vi "Create Channel Name Array.vi"(8 "error in":errorcluster, 9 "Number of Channels":u32=1, 10 "Channel Format String":string, 11 "Plugin Name":string) -> (0 "error out":errorcluster, 2 "Channel Names":string[](array[string]))   [LabVIEW 2023, in "Utilities.lvlib"]
uses:
  Utilities.lvlib
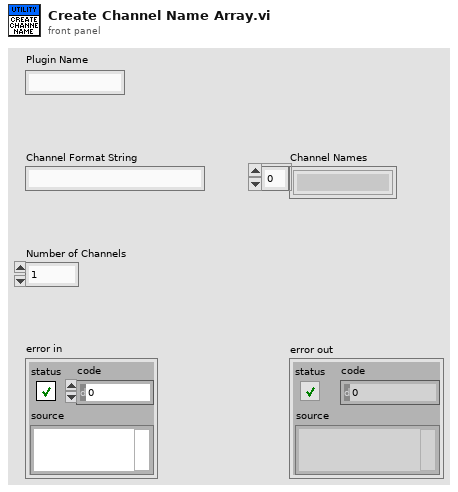
[diagram p1: front panel]
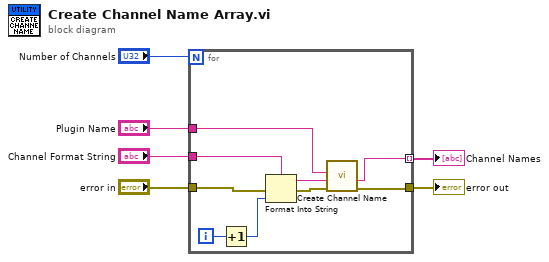
[diagram p0: block diagram]
diagram:
  n1 = for {
    N: "Number of Channels" -> [_]
    tunnel: [w14] -> w3
    tunnel: "Plugin Name" -> [w15]
    tunnel: "Channel Format String" -> [w12]
    tunnel: "error in" -> [w8]
    tunnel: [w7] -> w1 mode=indexing
    i -> [w11]
    n2 = Increment(x=w11) -> (x+1=w10:i32)
    n3 = Format Into String(format string=w12, error in=w8, w10) -> (resulting string=w13:string, error out=w9:errorcluster)  [unwired: 1 in]
    n4 = call "Create Channel Name.vi"("error in"=w9, "Channel Name"=w13, "Plugin Name"=w15) -> ("error out"=w14:errorcluster, "Data Channel Name"=w7:string)  [unwired: 7 in]
  }
  "error out" <- w3
  "Channel Names" <- w1
